vi "FilterShrouds.vi"(9 "Queue timeout (ms)":i32=200, 10 "NotifierReff 2":T1, 11 "Queue in":refnum<queue>) -> ()   [LabVIEW 2013]
doc: "Performs and filtering that we want (default is no filtering) and writes the data to the notifier. If no data is in the queue this VI times out after 'Queue timeout (ms)' has passed and nothing is written to the notifier.\n\nEric Schneider, March 2014"
uses:
  Data/TypeDefs/Notifiers.ctl
  Data/TypeDefs/UTM Location.ctl
  Data/TypeDefs/Sail Set Suggestions.ctl
  Data/TypeDefs/Rudder Set Suggestions.ctl
  Data/TypeDefs/OverrideInformation.ctl
  Data/TypeDefs/OverrideMode.ctl
  Data/TypeDefs/MotorSetup.ctl
  Data/TypeDefs/DynamixelSetupInfo.ctl
  Data/TypeDefs/AirmarStatus.ctl
  Data/TypeDefs/HardwareOnline.ctl
  Data/TypeDefs/DynamixelCycleTracker.ctl
  Data/TypeDefs/RC Input Values.ctl
  Classes/Missions/GenericMission/GenericMission.lvclass
  Classes/Waypoint/Waypoint.lvclass
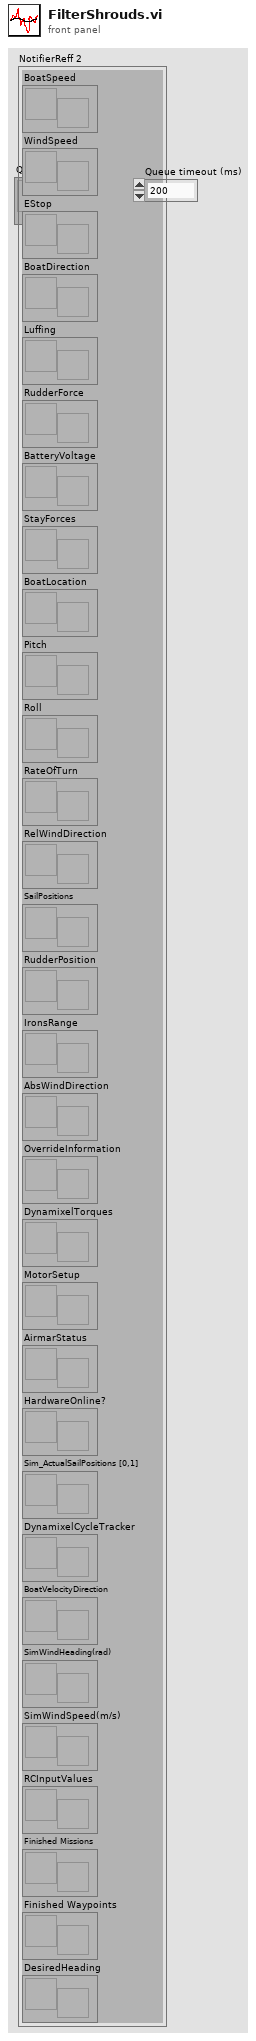
[diagram p1: front panel]
types:
  T1 = typedef "Notifiers.ctl" = cluster{"BoatSpeed":refnum<notifier>, "WindSpeed":refnum<notifier>, "EStop":refnum<notifier>, "BoatDirection":refnum<notifier>, "Luffing":refnum<notifier>, "RudderForce":refnum<notifier>, "BatteryVoltage":refnum<notifier>, "StayForces":refnum<notifier>, "BoatLocation":refnum<notifier>, "Pitch":refnum<notifier>, "Roll":refnum<notifier>, "RateOfTurn":refnum<notifier>, "RelWindDirection":refnum<notifier>, "SailPositions":refnum<notifier>, "RudderPosition":refnum<notifier>, "IronsRange":refnum<notifier>, "AbsWindDirection":refnum<notifier>, "OverrideInformation":refnum<notifier>, "DynamixelTorques":refnum<notifier>, "MotorSetup":refnum<notifier>, "AirmarStatus":refnum<notifier>, "HardwareOnline?":refnum<notifier>, "Sim_ActualSailPositions [0,1]":refnum<notifier>, "DynamixelCycleTracker":refnum<notifier>, "BoatVelocityDirection":refnum<notifier>, "SimWindHeading(rad)":refnum<notifier>, "SimWindSpeed(m/s)":refnum<notifier>, "RCInputValues":refnum<notifier>, "Finished Missions":refnum<notifier>, "Finished Waypoints":refnum<notifier>, "DesiredHeading":refnum<notifier>}
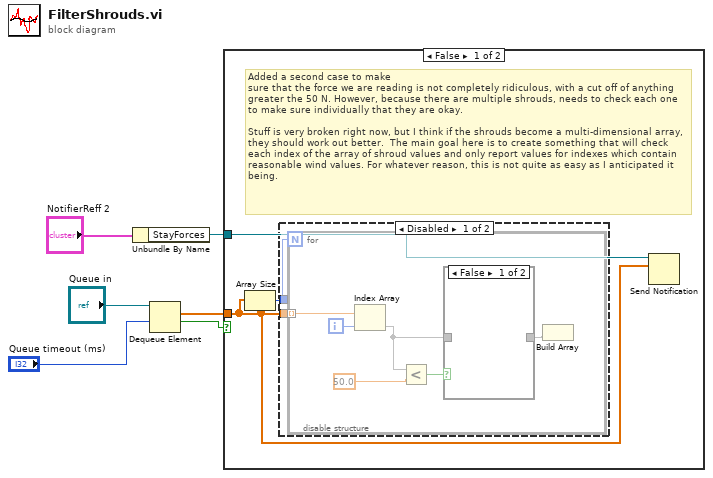
[diagram p0: block diagram]
diagram:
  n1 = Unbundle By Name("NotifierReff 2") -> ("StayForces"=w3:refnum<notifier>)
  n2 = Dequeue Element(queue="Queue in", timeout in ms (-1)="Queue timeout (ms)") -> (element=w5:dbl[], timed out?=w1:bool)  [unwired: 1 in, 2 out]
  n3 = case shown="False" w1 {
    tunnel: w5 -> [w7 _]
    tunnel: w3 -> [w9 _]
    frame False {
      # "Added a second case to make\nsure that the force we are reading is not completely ridiculous, with a cut off of anything greater the 50 N. However, because there are multiple shrouds, needs to check each one to make sure individually that they are okay.\n\nStuff is very broken right now, but I think if the shrouds become a multi-dimensional array, they should work out better.  The main goal here is to create something that will check each index of the array of shroud values and only report values for indexes which contain reasonable wind values. For whatever reason, this is not quite as easy as I anticipated it being."
      n4 = Array Size(array=w7) -> (size(s)=w8:i32)
      n5 = disable-structure shown="Disabled" {
        disable-tunnel: w8 -> [w11 _]
        disable-tunnel: w7 -> [w10 _]
        frame Disabled {
          n6 = for {
            N: w11 -> [_]
            tunnel: w10 -> [w16] mode=indexing
            i -> [w17]
            n7 = Index Array(array=w16, index=w17) -> (element=w13)
            n8 = Less?(x=w13, y=50.0) -> (x < y?=w15:bool)
            n9 = case shown="False" w15 {
              tunnel: w13 -> [_ w18]
              tunnel: [_ w18] -> w12
              frame False {
              }
              frame True {
              }
            }
            n10 = Build Array(w12) -> ()  [unwired: 1 in, 1 out]
          }
        }
        frame Enabled {
        }
      }
      n11 = Send Notification(notification=w7, notifier=w9) -> ()  [unwired: 1 in, 2 out]
    }
    frame True {
    }
  }
